vi "Reserve Sessions with Observer - Old.vi"(6 "timeout (ms)":i32, 7 "reservation observer":refnum<class "IReservationObserver.lvclass">, 8 "error in":errorcluster, 9 "instrument type id":string, 10 "pin or relay names":string[](array[string]), 11 "pin map context":T1) -> (0 "error out":errorcluster, 3 "session reservation out":refnum<class "Session Reservation.lvclass">)   [LabVIEW 2020, in "MeasurementLink Session Management.lvlib" / "Session Reservation.lvclass"]
uses:
  Session Reservation.lvclass
  Session Reservation.lvclass/Session Reservation.ctl
  MeasurementLink Session Management Client/RPC Messages/ni_measurementlink_PinMapContext.ctl
  MeasurementLink Session Management Client/MeasurementLink Session Management Client.lvlib
  MeasurementLink Session Management Client/RPC Messages/ni_measurementlink_sessionmanagement_v1_ReserveSessionsRequest.ctl
  MeasurementLink gRPC Utilities/gRPC Client Pool/gRPC Client Pool.lvclass
  MeasurementLink gRPC Utilities/gRPC Client Pool/FGV Action.ctl
  Data.ctl
  MeasurementLink Session Management Client/RPC Messages/ni_measurementlink_sessionmanagement_v1_SessionInformation.ctl
  MeasurementLink Session Management Client/RPC Messages/ni_measurementlink_sessionmanagement_v1_ChannelMapping.ctl
  MeasurementLink Session Management Client/RPC Messages/nidevice_grpc_Session.ctl
  Session and Driver Info.ctl
  Connection Map/Connection Map.lvclass
  MeasurementLink Instrument/IInstrument/IInstrument.lvclass
  IState/IState.lvclass
  Reserved State/Reserved State.lvclass
  IReservationObserver/IReservationObserver.lvclass
  \\tsclient\C/dev/measurementlink-labview/Source/Runtime/MeasurementLink Session Management/Reserved State/Reserved State.lvclass
  \\tsclient\C/dev/measurementlink-labview/Source/Runtime/MeasurementLink Session Management/IState/IState.lvclass
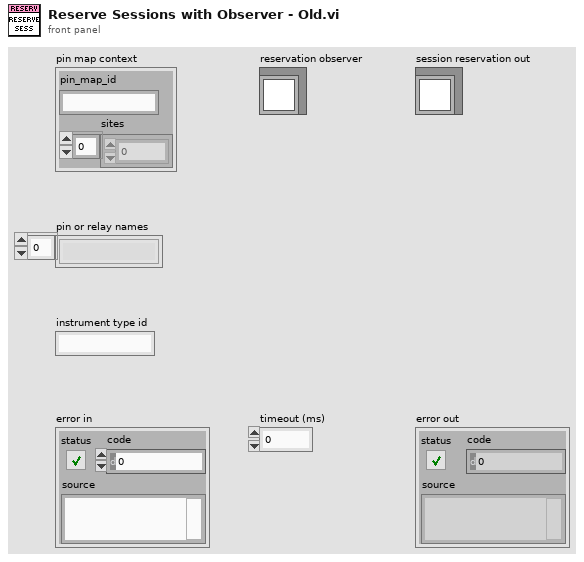
[diagram p1: front panel]
types:
  T1 = typedef "MeasurementLink Session Management Client.lvlib/ni_measurementlink_PinMapContext.ctl" = cluster{"pin_map_id":string, "sites":i32[]}
  T2 = typedef "MeasurementLink Session Management.lvlib/Session Reservation.lvclass/Data.ctl" = cluster{"session and driver infos":T3[], "pin or relay names":string[], "connection map":refnum<class "Connection Map.lvclass">, "pin map context":T1, "state":refnum<class "IState.lvclass">, "reservation observer":refnum<class "IReservationObserver.lvclass">}
  T3 = typedef "MeasurementLink Session Management.lvlib/Session Reservation.lvclass/Session and Driver Info.ctl" = cluster{"session info":T4, "session":variant, "instrument":refnum<class "IInstrument.lvclass">}
  T4 = typedef "MeasurementLink Session Management Client.lvlib/ni_measurementlink_sessionmanagement_v1_SessionInformation.ctl" = cluster{"session":T5, "resource_name":string, "channel_list":string, "instrument_type_id":string, "session_exists":bool, "channel_mappings":T6[]}
  T5 = typedef "MeasurementLink Session Management Client.lvlib/nidevice_grpc_Session.ctl" = cluster{"name":string}
  T6 = typedef "MeasurementLink Session Management Client.lvlib/ni_measurementlink_sessionmanagement_v1_ChannelMapping.ctl" = cluster{"pin_or_relay_name":string, "site":i32, "channel":string}
  T7 = typedef "MeasurementLink gRPC Utilities.lvlib/gRPC Client Pool.lvclass/FGV Action.ctl" = enum16{"Get Discovery Client", "Get Session Client", "Get Pinmap Client", "Destroy Clients"}
  T8 = typedef "MeasurementLink Session Management Client.lvlib/ni_measurementlink_sessionmanagement_v1_ReserveSessionsRequest.ctl" = cluster{"pin_map_context":T1, "pin_or_relay_names":string[], "instrument_type_id":string, "timeout_in_milliseconds":i32}
  T9 = typedef "grpc-lvsupport-release.lvlib/grpcId.ctl" = u64
  T10 = typedef "MeasurementLink Session Management Client.lvlib/ni_measurementlink_sessionmanagement_v1_ReserveSessionsResponse.ctl" = cluster{"sessions":T4[]}
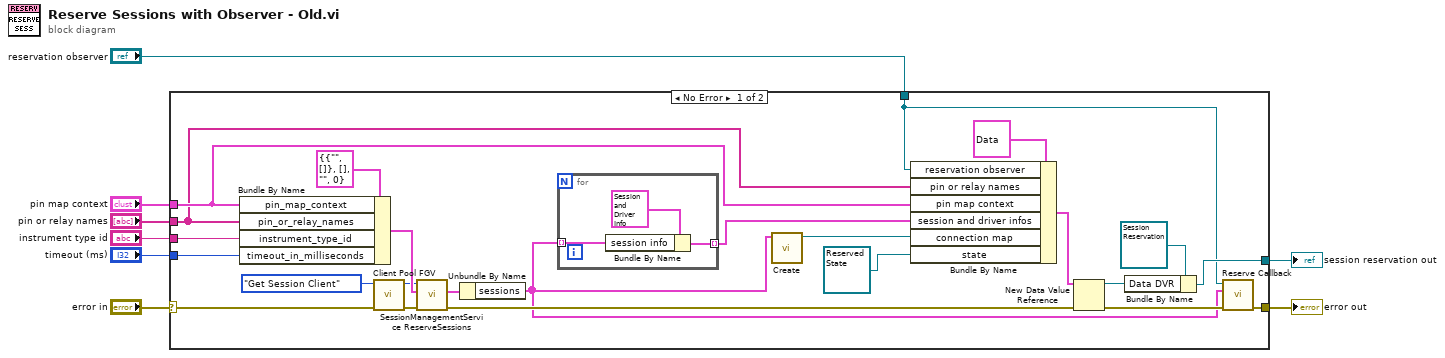
[diagram p0: block diagram]
diagram:
  n1 = case shown="No Error" "error in" {
    selector: "error in" -> [w23 w36]
    tunnel: "instrument type id" -> [w18 _]
    tunnel: "pin or relay names" -> [w13 _]
    tunnel: "timeout (ms)" -> [w17 _]
    tunnel: "pin map context" -> [w14 _]
    tunnel: [w26 _] -> w4
    tunnel: [w11 w36] -> w3
    tunnel: "reservation observer" -> [w10 _]
    frame No Error {
      n2 = Bundle By Name(cluster=T8 {"pin_map_context"={"pin_map_id"="", "sites"=[]}, "pin_or_relay_names"=[], "instrument_type_id"="", "timeout_in_milliseconds"=0} ("Request Data"), "pin_map_context"=w14, "pin_or_relay_names"=w13, "instrument_type_id"=w18, "timeout_in_milliseconds"=w17) -> (w31:T8)
      n3 = call "Client Pool FGV.vi"("error in (no error)"=w23, "Action"=FGV_Action."Get Session Client") -> ("error out"=w29:errorcluster, "grpc client id"=w28:T9)  [unwired: 8 in]
      n4 = call "SessionManagementService ReserveSessions.vi"("error in"=w29, "Request Data"=w31, "gRPC ID"=w28) -> ("error out"=w25:errorcluster, "Response Data"=w27:T10)  [unwired: 6 in, 1 out]
      n5 = Unbundle By Name(w27) -> ("sessions"=w9:T4[])
      n6 = for {
        tunnel: w9 -> [w35] mode=indexing
        tunnel: [w34] -> w15 mode=indexing
        n7 = Bundle By Name(cluster=T3 {"session info"={"session"={"name"=""}, "resource_name"="", "channel_list"="", "instrument_type_id"="", "session_exists"=FALSE, "channel_mappings"=[]}, "session"=variant, "instrument"=refnum} ("session and driver info"), "session info"=w35) -> (w34:T3)
      }
      n8 = call "Create.vi"("session info"=w9) -> ("connection map"=w16:refnum<class "Connection Map.lvclass">)  [unwired: 10 in]
      n9 = Bundle By Name(cluster=T2 {"session and driver infos"=[], "pin or relay names"=[], "connection map"=refnum, "pin map context"={"pin_map_id"="", "sites"=[]}, "state"=refnum, "reservation observer"=refnum} ("session reservation data"), "reservation observer"=w10, "pin or relay names"=w13, "pin map context"=w14, "session and driver infos"=w15, "connection map"=w16, "state"=refnum<class "Reserved State.lvclass"> refnum ("MeasurementLink Session Management.lvlib:Reserved State.lvclass")) -> (w21:T2)
      n10 = New Data Value Reference(data value=w21, error in=w25) -> (data value reference=w19:refnum<data-value>, error out=w24:errorcluster)
      n11 = Bundle By Name(cluster=refnum<class "Session Reservation.lvclass"> refnum ("session reservation"), "Data DVR"=w19) -> (w26:refnum<class "Session Reservation.lvclass">)
      n12 = call-dynamic "Reserve Callback.vi"("error in"=w24, "session infos"=w9, "reservation observer in"=w10) -> ("error out"=w11:errorcluster)  [unwired: 7 in, 1 out]
    }
    frame Error {
    }
  }
  "session reservation out" <- w4
  "error out" <- w3
